vi "Create Data Channel - Single Channel - Format.vi"(8 "error in (no error)":errorcluster, 9 "settings":T1, 10 "channel name":string, 11 "response refnum in":T2 format="%.0x") -> (0 "error out":errorcluster, 2 "channel refnum":T2 format="%.0x", 3 "response refnum out":T2 format="%.0x")   [LabVIEW 2020, in "Instrument Addon Scripting API.lvlib"]
doc: "Creates a new Data Channel under the specified response."
uses:
  Instrument Addon Scripting API.lvlib
  <vilib>/NI VeriStand/Custom Device API/Custom Device Item Ref.ctl
  TypeDefs/Single Channel Format Settings.ctl
  Shared Directory/Data Parameters.ctl
  Shared Directory/Protocol Data Type.ctl
  Shared Directory/Data Channel Type.ctl
  Shared Directory/Type Cast Type.ctl
  Shared Directory/Endian.ctl
  <vilib>/NI VeriStand/Custom Device API/Custom Device Channel.ctl
  <vilib>/NI VeriStand/Custom Device API/Custom Device Channel Type.ctl
  Shared Directory/Instrument Addon Shared.lvlib
  <vilib>/NI VeriStand/Custom Device API/Custom Device API.lvlib
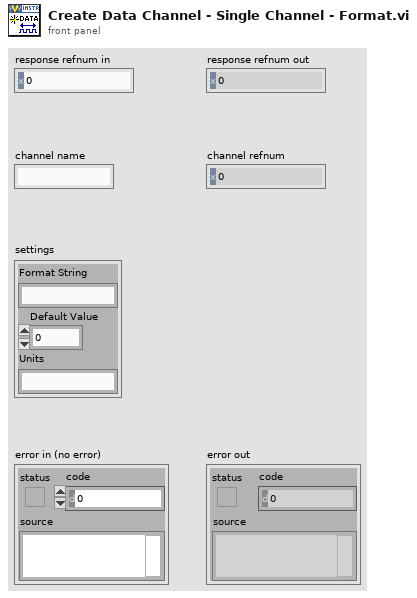
[diagram p1: front panel]
types:
  T1 = typedef "Instrument Addon Scripting API.lvlib/Single Channel Format Settings.ctl" = cluster{"Format String":string, "Default Value":dbl, "Units":string}
  T2 = typedef "Custom Device API.lvlib/Custom Device Item Ref.ctl" = u64
  T3 = typedef "Instrument Addon Shared.lvlib/Data Channel Type.ctl" = enum16{"Format", "Comparison", "Type Cast", "Enumerated List"}
  T4 = typedef "Instrument Addon Shared.lvlib/Protocol Data Type.ctl" = enum16{"Single Channel", "Array"}
  T5 = typedef "Custom Device API.lvlib/Custom Device Channel.ctl" = cluster{"Type":T6, "Units":string, "Default Value":dbl, "Faultable":bool, "Scalable":bool}
  T6 = typedef "Custom Device API.lvlib/Custom Device Channel Type.ctl" = enum16{"Input", "Output"}
  T7 = typedef "Instrument Addon Shared.lvlib/Data Parameters.ctl" = cluster{"Data Type":T4, "Channel Type":T3, "Format String":string, "Expected String":string, "Type":T8, "List":string[], "Delimiter":string, "Endian":T9}
  T8 = typedef "Instrument Addon Shared.lvlib/Type Cast Type.ctl" = enum16{"DBL", "SGL", "U64", "U32", "U16", "U8", "I64", "I32", "I16", "I8"}
  T9 = typedef "Instrument Addon Shared.lvlib/Endian.ctl" = enum16{"Native", "Little", "Big"}
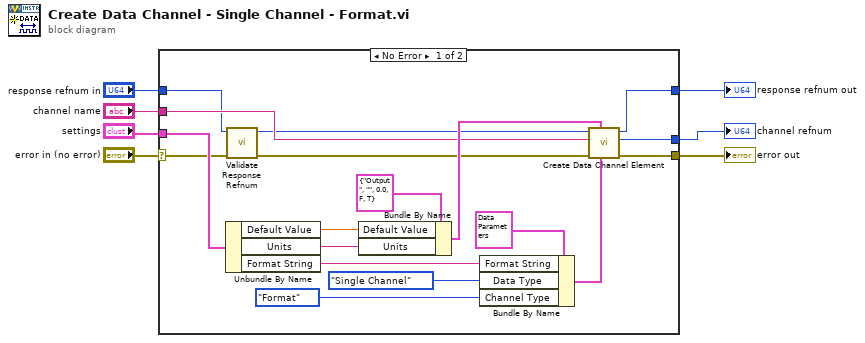
[diagram p0: block diagram]
diagram:
  n1 = case shown="No Error" "error in (no error)" {
    selector: "error in (no error)" -> [w11 w27]
    tunnel: [w17 w27] -> w7
    tunnel: [w13 w26] -> w6
    tunnel: [w16 _] -> w5
    tunnel: "channel name" -> [w12 _]
    tunnel: "response refnum in" -> [w9 w26]
    tunnel: "settings" -> [w21 _]
    frame No Error {
      n2 = Unbundle By Name(w21) -> ("Default Value"=w23:dbl, "Units"=w22:string, "Format String"=w20:string)
      n3 = call "Validate Response Refnum.vi"("error in (no error)"=w11, "response refnum in"=w9) -> ("error out"=w10:errorcluster, "response refnum out"=w8:u64)  [unwired: 8 in]
      n4 = Bundle By Name(cluster=T5 {"Type"=enum."Output", "Units"="", "Default Value"=0.0, "Faultable"=FALSE, "Scalable"=TRUE} ("Channel"), "Default Value"=w23, "Units"=w22) -> (w14:T5)
      n5 = Bundle By Name(cluster=T7 {"Data Type"=enum."Single Channel", "Channel Type"=enum."Format", "Format String"="%.3g", "Expected String"="", "Type"=enum."SGL", "List"=[], "Delimiter"=",", "Endian"=enum."Native"} ("Data Parameters"), "Format String"=w20, "Data Type"=Protocol_Data_Type."Single Channel", "Channel Type"=Data_Channel_Type."Format") -> (w15:T7)
      n6 = call "Create Data Channel Element.vi"("Data Channel Parameters"=w15, "Settings"=w14, "Error In"=w10, "Name"=w12, "Refnum In"=w8) -> ("Error Out"=w17:errorcluster, "Channel Refnum"=w16:T2, "Refnum Out"=w13:T2)  [unwired: 4 in]
    }
    frame Error {
    }
  }
  "error out" <- w7
  "response refnum out" <- w6
  "channel refnum" <- w5
